vi "set Power-on Status Clear.vi"(8 "error in (no error)":errorcluster, 10 "PSC Flag (false)":bool, 11 "VISA resource name":refnum<visa-resource-name>) -> (0 "error out":errorcluster, 3 "VISA resource name out":refnum<visa-resource-name>, 4 "Device Errors":cluster{"code":i32, "Text":string}[](array[cluster]))   [LabVIEW 2014, in "Stanford Research DG645 - Driver.lvlib"]
doc: "Common IEEE-488.2 Command: *PSC i\nInstrument Error Check\n\nSet the Power-on Status Clear flag to true (1) or false (0). The Power-on Status Clear flag is stored in nonvolontile memory in the DG645, and thus, maintains its value through power-cycle events. \n\nIf the value on the flag is false, then the Service Request Enable and Standard Event Status Enable Registers (*SRE, *ESE) are stored in non-volontile memory, and retain their values through power-cycle events. If the value of the flag is true, then these two registers are cleared upon power-cycle."
uses:
  Stanford Research DG645 - Driver.lvlib
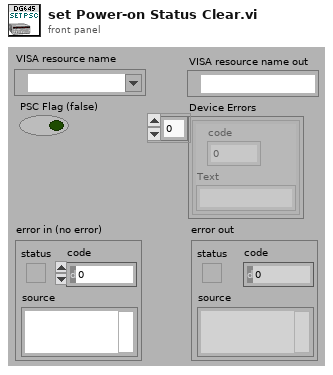
[diagram p1: front panel]
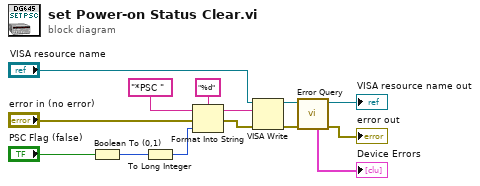
[diagram p0: block diagram]
diagram:
  n1 = Boolean To (0,1)(Boolean="PSC Flag (false)") -> (0, 1=w2:i16)
  n2 = To Long Integer(number=w2) -> (32bit integer=w1:i32)
  n3 = Format Into String(format string="%d", initial string="*PSC " ("command"), error in="error in (no error)", w1) -> (resulting string=w5:string, error out=w3:errorcluster)
  n4 = VISA Write(VISA resource name="VISA resource name", write buffer=w5, error in (no error)=w3) -> (VISA resource name out=w11:refnum<visa-resource-name>, error out=w13:errorcluster)  [unwired: 1 out]
  n5 = call "Error Query.vi"("error in (no error)"=w13, "VISA resource name"=w11) -> ("error out"=→"error out":errorcluster, "VISA resource name out"=→"VISA resource name out":refnum<visa-resource-name>, "Device Errors"=→"Device Errors":cluster{"code":i32, "Text":string}[])  [unwired: 7 in]
